vi "behavior_only_with_reward_shaping.vi"() -> ()   [LabVIEW 2019]
doc: "The myRIO Project template acquires acceleration data from the onboard accelerometer and displays the changes of acceleration values in a waveform chart."
uses:
  <vilib>/myRIO/Common/Instrument Driver Framework/myRIO v1.0/Encoder/typedefs/Encoder Signal Mode.ctl
  <vilib>/myRIO/Instrument Drivers/Onboard IO/Encoder/typedefs/Encoder Reference.ctl
  <vilib>/myRIO/Common/Instrument Driver Framework/Utilities/typedefs/myRIO Generic Hardware Reference.ctl
  <vilib>/myRIO/Common/Instrument Driver Framework/Utilities/typedefs/Hardware Version Enum.ctl
  <vilib>/myRIO/Common/Instrument Driver Framework/Utilities/typedefs/myRIO v1.0 Reference.ctl
  <vilib>/myRIO/Common/Instrument Driver Framework/Utilities/typedefs/Generic FPGA Reference.ctl
  <vilib>/myRIO/Common/Instrument Driver Framework/myRIO v1.0/Encoder/typedefs/Encoder Channels Enum.ctl
  <vilib>/myRIO/Common/Instrument Driver Framework/myRIO v1.0/Encoder/typedefs/Encoder Configuration v1.0.ctl
  <vilib>/userdefined/High Color/nirio_resource_hc.ctl
  <vilib>/myRIO/Instrument Drivers/Onboard IO/DIO/typedefs/DIO Reference.ctl
  <vilib>/myRIO/Common/Instrument Driver Framework/myRIO v1.0/DIO/typedefs/DIO Channels List.ctl
  <vilib>/myRIO/Common/Instrument Driver Framework/myRIO v1.0/DIO/typedefs/DIO Channels Enum.ctl
  <vilib>/myRIO/Common/Instrument Driver Framework/Utilities/vis/Is FPGA Ref Available.vi
  <vilib>/myRIO/Common/Instrument Driver Framework/myRIO v1.0/Encoder/vis/myRIO v1.1 Open Encoder.vi
  <vilib>/myRIO/Instrument Drivers/Onboard IO/Encoder/vis/Read.vi
  <vilib>/myRIO/Common/Instrument Driver Framework/myRIO v1.0/DIO/vis/myRIO v1.1 Open DIO.vi
  <vilib>/myRIO/Instrument Drivers/Onboard IO/DIO/vis/Read.vi
  <vilib>/myRIO/Instrument Drivers/Onboard IO/DIO/vis/Write.vi
  <vilib>/myRIO/Common/Instrument Driver Framework/Utilities/vis/Validate Channels.vi
  <vilib>/myRIO/Common/Instrument Driver Framework/myRIO v1.0/Encoder/vis/myRIO v1.0 Reserve Encoder.vi
  <vilib>/myRIO/Common/Instrument Driver Framework/myRIO v1.0/DIO/vis/myRIO v1.0 Reserve DIO.vi
  <vilib>/myRIO/Common/Instrument Driver Framework/myRIO v1.0/Encoder/vis/myRIO v1.0 Build MUX Configuration Encoder.vi
  <vilib>/myRIO/Common/Instrument Driver Framework/myRIO v1.0/Resource Manager/vis/myRIO v1.0 Reserve Channel List.vi
  <vilib>/myRIO/Common/Instrument Driver Framework/myRIO v1.0/DIO/vis/myRIO v1.0 Build MUX Configuration DIO.vi
  <vilib>/myRIO/Common/Instrument Driver Framework/myRIO v1.0/Resource Manager/vis/myRIO v1.0 Create Configuration List.vi
  <vilib>/myRIO/Common/Instrument Driver Framework/myRIO v1.0/Resource Manager/vis/myRIO v1.0 Reserve Channel.vi
  <vilib>/myRIO/Common/Instrument Driver Framework/myRIO v1.0/Resource Manager/vis/myRIO v1.0 Unreserve Channel.vi
  <vilib>/myRIO/Common/Instrument Driver Framework/myRIO v1.0/Resource Manager/vis/myRIO v1.0 Build Mutex Name.vi
  <vilib>/Utility/VariantDataType/GetNumericInfo.vi
  <vilib>/Utility/error.llb/Error Cluster From Error Code.vi
  <vilib>/myRIO/Common/Instrument Driver Framework/myRIO v1.0/myRIO v1.1 Open.vi
  <vilib>/myRIO/Common/Instrument Driver Framework/Utilities/vis/IO Manager.vi
  <vilib>/myRIO/Common/Instrument Driver Framework/Utilities/vis/Configuration Manager.vi
  <vilib>/myRIO/Common/Instrument Driver Framework/myRIO v1.0/Resource Manager/vis/myRIO v1.0 Configure IO.vi
  <vilib>/myRIO/Common/Instrument Driver Framework/myRIO v1.0/myRIO v1.0 Close.vi
  <vilib>/myRIO/Common/Instrument Driver Framework/myRIO v1.0/Encoder/vis/myRIO v1.0 Configure Encoder.vi
  <vilib>/myRIO/Common/Instrument Driver Framework/myRIO v1.0/Encoder/vis/myRIO v1.0 Read Encoder.vi
  <vilib>/myRIO/Common/Instrument Driver Framework/myRIO v1.0/DIO/vis/myRIO v1.0 Read DIO.vi
  <vilib>/myRIO/Common/Instrument Driver Framework/myRIO v1.0/DIO/vis/myRIO v1.0 Write DIO.vi
  <vilib>/myRIO/Express VI/Onboard IO/Encoder/Encoder Express VI.xnode
  <vilib>/myRIO/Instrument Drivers/Onboard IO/Encoder/vis/myRIO Encoder Open.xnode
  <vilib>/myRIO/Express VI/Onboard IO/DI/DI Express VI.xnode
  <vilib>/myRIO/Instrument Drivers/Onboard IO/DIO/vis/myRIO DIO Open.xnode
  <vilib>/myRIO/Express VI/Onboard IO/DO/DO Express VI.xnode
  <vilib>/myRIO/Instrument Drivers/Onboard IO/Encoder/Encoder.lvlib
  <vilib>/myRIO/Instrument Drivers/Onboard IO/DIO/DIO.lvlib
panel:
  out "Frame clock":i32
  out "Frames":u32
  out "Reward":bool=TRUE
  in  "Give reward":bool
  out "Licks":u32
  out "Lick":bool
  out "Output":dbl[][](array[numeric])
  out "Time":dbl
  out "Display":bool
  out "Stop":bool
  in  "Frames to collect":u32
  out "Overflow?":bool
  out "Counter Value":i32
  out "Velocity":dbl
  out "Velocity Plot":dbl[](graph)
  out "Velocity array":dbl[](array[numeric])
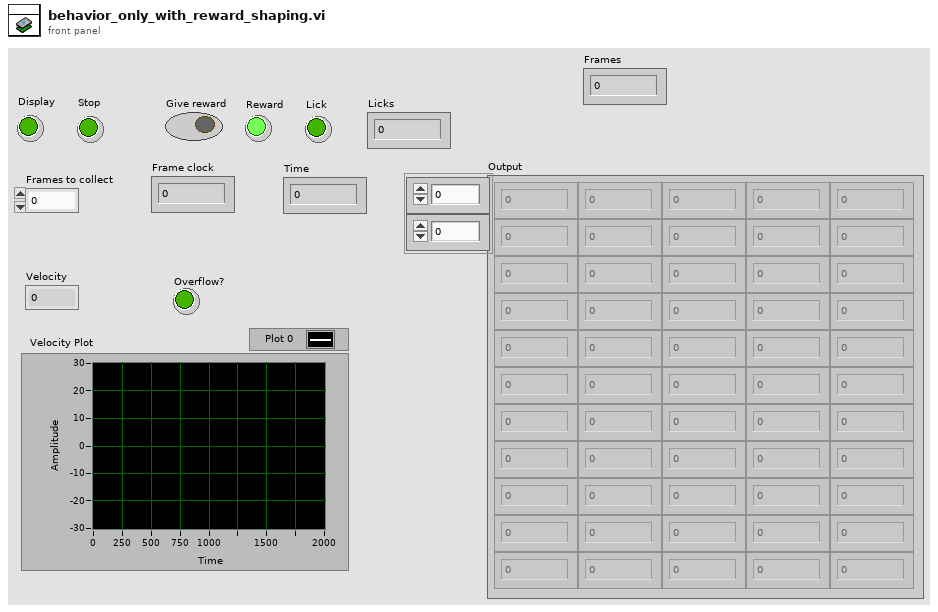
[diagram p1: front panel]
types:
  T1 = typedef "Encoder.lvlib/Encoder Reference.ctl" = cluster{"myRIO Reference":T2, "Encoder Channels Enum":T6}
  T2 = typedef "myRIO Generic Hardware Reference.ctl" = cluster{"myRIO Model":T3, "myRIO Hardware Reference":T4}
  T3 = typedef "Hardware Version Enum.ctl" = enum16{"Unknown", "myRIO-1900", "myRIO-1950", "roboRIO", "NI ELVIS RIO CM", "ELVIS III"}
  T4 = typedef "myRIO v1.0 Reference.ctl" = cluster{"Generic FPGA Reference":T5, "Allow multiple opens":bool}
  T5 = typedef "Generic FPGA Reference.ctl" = refnum<k20>
  T6 = typedef "Encoder Channels Enum.ctl" = enum16{"Not Connected", "C/ENC0", "C/ENC1", "A/ENC", "A/ENC0", "A/ENC1", "A/ENC2", "A/ENC3", "A/ENC4", "A/ENC5", "A/ENC6", "A/ENC7", "A/ENC8", "A/ENC9", "B/ENC", "B/ENC0", "B/ENC1", "B/ENC2", "B/ENC3", "B/ENC4", "B/ENC5", "B/ENC6", "B/ENC7", "B/ENC8", "B/ENC9", "DIO/ENC0", "DIO/ENC1", "DIO/ENC2", "DIO/ENC3", "DIO/ENC4"}
  T7 = typedef "Encoder Signal Mode.ctl" = enum16{"Quadrature phase signal", "Step and direction signal"}
  T8 = typedef "nirio_resource_hc.ctl" = tag
  T9 = typedef "DIO.lvlib/DIO Reference.ctl" = cluster{"myRIO Reference":T2, "DIO Channels List":T10}
  T10 = typedef "DIO Channels List.ctl" = T11[]
  T11 = typedef "DIO Channels Enum.ctl" = enum16{"Not Connected", "C/DIO0", "C/DIO1", "C/DIO2", "C/DIO3", "C/DIO4", "C/DIO5", "C/DIO6", "C/DIO7", "A/DIO0", "A/DIO1", "A/DIO2", "A/DIO3", "A/DIO4", "A/DIO5", "A/DIO6", "A/DIO7", "A/DIO8", "A/DIO9", "A/DIO10", "A/DIO11", "A/DIO12", "A/DIO13", "A/DIO14", "A/DIO15", "A/DIO16", "A/DIO17", "A/DIO18", "A/DIO19", "B/DIO0", "B/DIO1", "B/DIO2", "B/DIO3", "B/DIO4", "B/DIO5", "B/DIO6", "B/DIO7", "B/DIO8", "B/DIO9", "B/DIO10", "B/DIO11", "B/DIO12", "B/DIO13", "B/DIO14", "B/DIO15", "B/DIO16", "B/DIO17", "B/DIO18", "B/DIO19", "LED0", "LED1", "LED2", "LED3", "Button0", "DIO/DIO0", "DIO/DIO1", "DIO/DIO2", "DIO/DIO3", "DIO/DIO4", "DIO/DIO5", "DIO/DIO6", "DIO/DIO7", "DIO/DIO8", "DIO/DIO9", "SPI/CS0", "SPI/CS1", "SPI/CS2", "SPI/CS3", "LED RADIO (Green)", "LED RADIO (Red)", "LED COMM (Green)", "LED COMM (Red)", "LED MODE (Green)", "LED MODE (Red)"}
  T12 = typedef "NI_Matrix.lvlib/RealMatrix.ctl" = dbl[][]
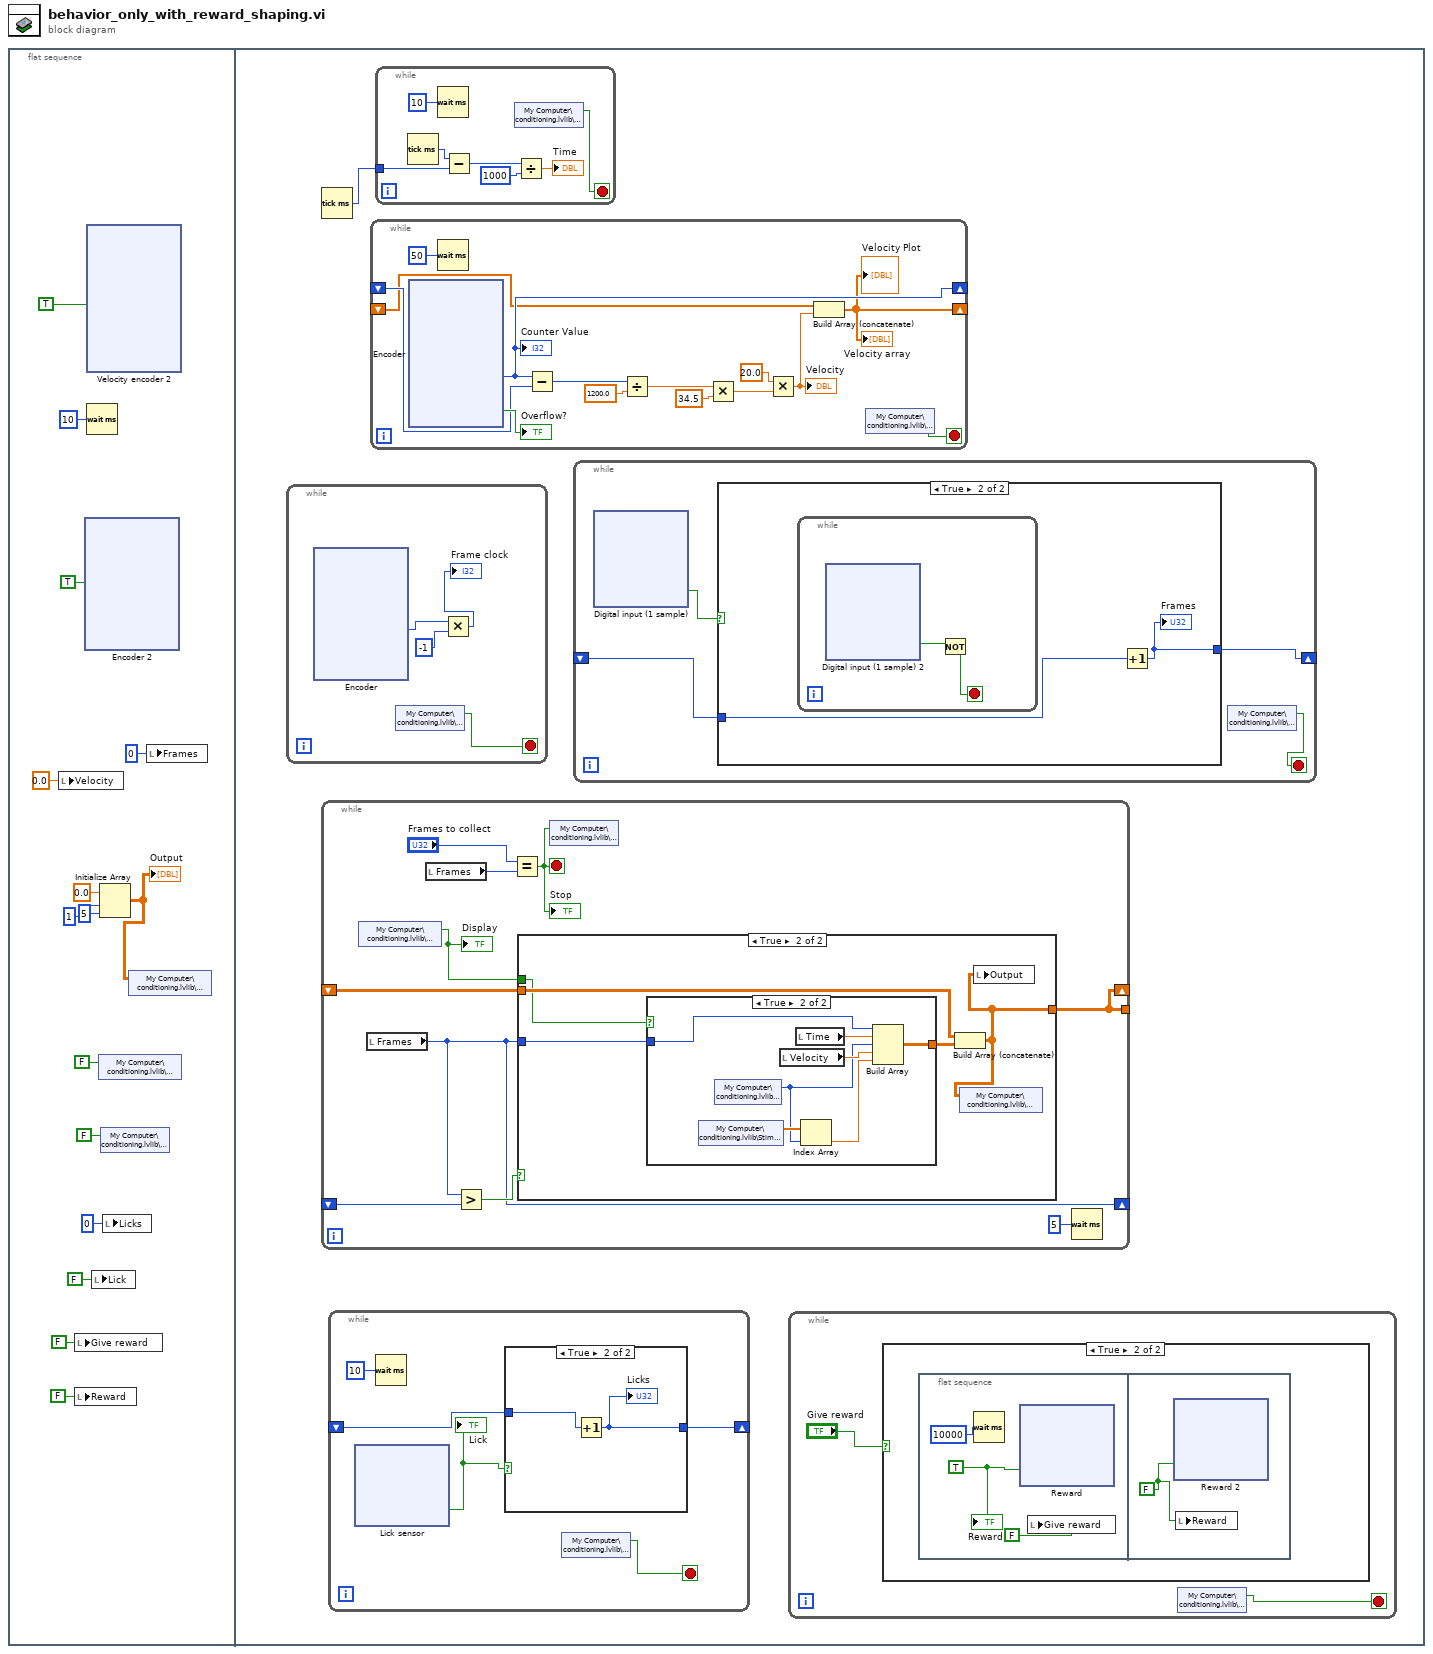
[diagram p0: block diagram]
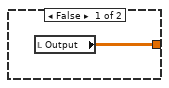
[diagram p5: hidden frame]
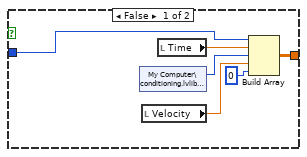
[diagram p6: hidden frame]
diagram:
  n1 = flat-sequence {
    frame #0 {
      n2 = local write "Velocity"(0.0 ("Velocity")) -> ()
      n3 = local write "Give reward"(FALSE ("Give reward")) -> ()
      n4 = local write "Reward"(FALSE ("Reward")) -> ()
      n5 = xnode "Encoder 2"("Reset Counter"=TRUE) -> ()  [unwired: 1 in, 4 out]
      n6 = xnode "Velocity encoder 2"("Reset Counter"=TRUE) -> ()  [unwired: 1 in, 4 out]
      n7 = Wait (ms)(milliseconds to wait=u32 10) -> ()  [unwired: 1 out]
      n8 = local write "Lick"(FALSE ("Lick")) -> ()
      n9 = shared-variable "My Computer\\conditioning.lvlib\\Display"(FALSE ("Display")) -> ()  [unwired: 1 in, 1 out]
      n10 = Initialize Array(0.0 ("element"), 1 ("dimension size"), 5 ("dimension size")) -> (w9:dbl[][])
      "Output" <- w9
      n11 = shared-variable "My Computer\\conditioning.lvlib\\Stop"(FALSE ("Stop")) -> ()  [unwired: 1 in, 1 out]
      n12 = local write "Licks"(u32 0 ("Licks")) -> ()
      n13 = shared-variable "My Computer\\conditioning.lvlib\\Output"(w9) -> ()  [unwired: 1 in, 1 out]
      n14 = local write "Frames"(u32 0 ("Frames")) -> ()
    }
    frame #1 {
      n15 = while {
        stop <- w109 stop-if-true
        n16 = xnode "Encoder"() -> ("Counter Value"=w112:i32)  [unwired: 2 in, 3 out]
        n17 = shared-variable "My Computer\\conditioning.lvlib\\Stop"() -> (w109:bool)  [unwired: 1 in, 1 out]
        n18 = Multiply(x=w112, y=-1) -> (x*y=→"Frame clock":i32)
      }
      n19 = Tick Count (ms)() -> (millisecond timer value=w108:u32)
      n20 = while {
        shift-right: [w431] -> _
        shift-left: _ -> [w433]
        shift-right: [w426] -> _
        shift-left: _ -> [w430]
        tunnel: [w426] -> _
        stop <- w425 stop-if-true
        n21 = shared-variable "My Computer\\conditioning.lvlib\\Display"() -> (w424:bool)  [unwired: 1 in, 1 out]
        "Display" <- w424
        n22 = local read "Frames"() -> (w431:u32)
        n23 = local read "Frames"() -> (w428:u32)
        n24 = Greater?(x=w431, y=w433) -> (0:w432:bool)
        n25 = Equal?(x="Frames to collect", y=w428) -> (x = y?=w425:bool)
        "Stop" <- w425
        n26 = case shown="True" w432 {
          tunnel: w431 -> [_ w439]
          tunnel: w430 -> [_ w438]
          tunnel: [w434 w435] -> w426
          tunnel: w424 -> [_ w436]
          frame False {
            n27 = local read "Output"() -> (w434:dbl[][])
          }
          frame True {
            n28 = case shown="True" w436 {
              tunnel: w439 -> [w440 w452]
              tunnel: [w444 w451] -> w437
              frame False {
                n29 = shared-variable "My Computer\\conditioning.lvlib\\Trial"() -> (w442:u32)  [unwired: 1 in, 1 out]
                n30 = local read "Velocity"() -> (w441:dbl)
                n31 = local read "Time"() -> (w443:dbl)
                n32 = Build Array(w440, w443, w442, w441, 0) -> (w444:T12)
              }
              frame True {
                n33 = shared-variable "My Computer\\conditioning.lvlib\\Stim_ID"() -> (w448:dbl[])  [unwired: 1 in, 1 out]
                n34 = shared-variable "My Computer\\conditioning.lvlib\\Trial"() -> (w447:u32)  [unwired: 1 in, 1 out]
                n35 = local read "Velocity"() -> (w449:dbl)
                n36 = local read "Time"() -> (w450:dbl)
                n37 = Index Array(array=w448, index=w447) -> (element=w446:dbl)
                n38 = Build Array(w452, w450, w447, w449, w446) -> (w451:T12)
              }
            }
            n39 = Build Array (concatenate)(w438, w437) -> (w435:T12)
            n40 = shared-variable "My Computer\\conditioning.lvlib\\Output"(w435) -> ()  [unwired: 1 in, 1 out]
            n41 = local write "Output"(w435) -> ()
          }
        }
        n42 = shared-variable "My Computer\\conditioning.lvlib\\Stop"(w425) -> ()  [unwired: 1 in, 1 out]
        n43 = Wait (ms)(milliseconds to wait=u32 5) -> ()  [unwired: 1 out]
      }
      n44 = while {
        shift-right: [w315] -> _
        shift-left: _ -> [w314]
        stop <- w318 stop-if-true
        n45 = xnode "Lick sensor"() -> ("C/DIO1 (DIO1)"=w316:bool)  [unwired: 1 in, 1 out]
        "Lick" <- w316
        n46 = Wait (ms)(milliseconds to wait=u32 10) -> ()  [unwired: 1 out]
        n47 = case shown="True" w316 {
          tunnel: [w319 w321] -> w315
          tunnel: w314 -> [w319 w320]
          frame False {
          }
          frame True {
            n48 = Increment(x=w320) -> (x+1=w321:u32)
            "Licks" <- w321
          }
        }
        n49 = shared-variable "My Computer\\conditioning.lvlib\\Stop"() -> (w318:bool)  [unwired: 1 in, 1 out]
      }
      n50 = while {
        shift-right: [w367] -> _
        shift-left: _ -> [w368]
        shift-right: [w359] -> _
        shift-left: _ -> [w358]
        stop <- w357 stop-if-true
        n51 = xnode "Encoder"() -> ("Counter Value"=w367:i32, "Overflow?"=→"Overflow?":bool)  [unwired: 2 in, 2 out]
        "Counter Value" <- w367
        n52 = Wait (ms)(milliseconds to wait=u32 50) -> ()  [unwired: 1 out]
        n53 = Subtract(x=w367, y=w368) -> (x-y=w360:i32)
        n54 = Divide(x=w360, y=1200.0 ("600")) -> (x/y=w365:dbl)
        n55 = Multiply(x=w365, y=34.5) -> (x*y=w363:dbl)
        n56 = Multiply(x=20.0, y=w363) -> (x*y=w361:dbl)
        "Velocity" <- w361
        n57 = Build Array (concatenate)(w358, w361) -> (w359:dbl[])
        "Velocity Plot" <- w359
        "Velocity array" <- w359
        n58 = shared-variable "My Computer\\conditioning.lvlib\\Stop"() -> (w357:bool)  [unwired: 1 in, 1 out]
      }
      n59 = while {
        tunnel: w108 -> [w422]
        stop <- w417 stop-if-true
        n60 = Tick Count (ms)() -> (millisecond timer value=w423:u32)
        n61 = Wait (ms)(milliseconds to wait=u32 10) -> ()  [unwired: 1 out]
        n62 = Subtract(x=w423, y=w422) -> (x-y=w420:u32)
        n63 = shared-variable "My Computer\\conditioning.lvlib\\Stop"() -> (w417:bool)  [unwired: 1 in, 1 out]
        n64 = Divide(x=w420, y=u32 1000) -> (x/y=→"Time":dbl)
      }
      n65 = while {
        shift-right: [w162] -> _
        shift-left: _ -> [w161]
        stop <- w160 stop-if-true
        n66 = xnode "Digital input (1 sample)"() -> ("A/DIO13 (Pin 26)"=w159:bool)  [unwired: 1 in, 1 out]
        n67 = case shown="True" w159 {
          tunnel: [w198 w200] -> w162
          tunnel: w161 -> [w198 w199]
          frame False {
          }
          frame True {
            n68 = while {
              stop <- w202 stop-if-true
              n69 = xnode "Digital input (1 sample) 2"() -> ("A/DIO13 (Pin 26)"=w201:bool)  [unwired: 1 in, 1 out]
              n70 = Not(x=w201) -> (.not. x?=w202:bool)
            }
            n71 = Increment(x=w199) -> (x+1=w200:u32)
            "Frames" <- w200
          }
        }
        n72 = shared-variable "My Computer\\conditioning.lvlib\\Stop"() -> (w160:bool)  [unwired: 1 in, 1 out]
      }
      n73 = while {
        stop <- w238 stop-if-true
        n74 = case shown="True" "Give reward" {
          frame False {
          }
          frame True {
            n75 = flat-sequence {
              frame #0 {
                w242 = TRUE ("C/DIO0 (DIO0)")
                n76 = Wait (ms)(milliseconds to wait=u32 10000) -> ()  [unwired: 1 out]
                n77 = xnode "Reward"("C/DIO0 (DIO0)"=w242) -> ()  [unwired: 1 in, 1 out]
                n78 = local write "Give reward"(FALSE ("Give reward")) -> ()
                "Reward" <- w242
              }
              frame #1 {
                w278 = FALSE ("C/DIO0 (DIO0)")
                n79 = xnode "Reward 2"("C/DIO0 (DIO0)"=w278) -> ()  [unwired: 1 in, 1 out]
                n80 = local write "Reward"(w278) -> ()
              }
            }
          }
        }
        n81 = shared-variable "My Computer\\conditioning.lvlib\\Stop"() -> (w238:bool)  [unwired: 1 in, 1 out]
      }
    }
  }
